vi "CAN Reset.vi"(8 "错误输入（无错误）":errorcluster, 11 "Channel in":u16) -> (0 "错误输出":errorcluster, 2 "Channel out":u16, 3 "function return":u32)   [LabVIEW 2021, in "PCANBasic.lvlib"]
doc: "TPCANStatus __stdcall CAN_Reset(\n TPCANHandle Channel);"
uses:
  <userlib>/PCANBasic/PCANBasic.lvlib
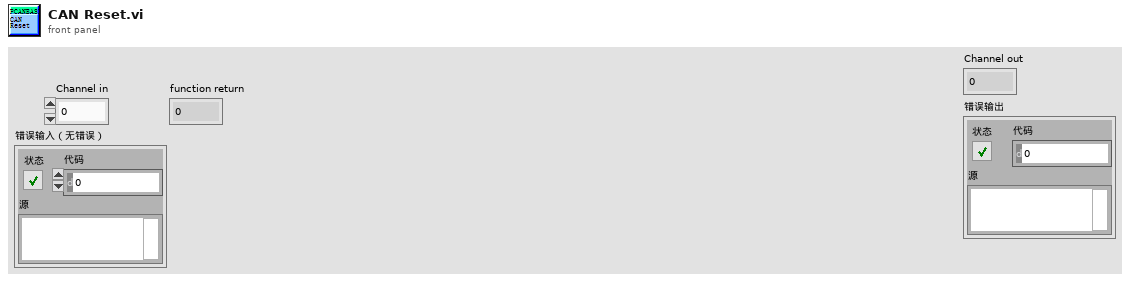
[diagram p1: front panel]
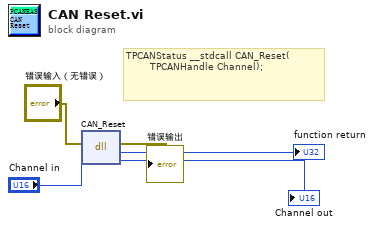
[diagram p0: block diagram]
diagram:
  # "TPCANStatus __stdcall CAN_Reset(\n        TPCANHandle Channel);"
  n1 = dll-call lib="PTH2gabs CUsersAdministrator.CH-202202160008Desktop电流传感器测试\tdll文件\nPCANBasic.dll" fn="CAN_Reset"(error in="错误输入（无错误）", "Channel"="Channel in") -> (error out=→"错误输出":errorcluster, "返回类型"=→"function return":u32, "Channel"=→"Channel out":u16)  [unwired: 2 in, 1 out]
